vi "example.vi"() -> ()   [LabVIEW 2019]
panel:
  in  "Input Potentials":dbl[](array[numeric])
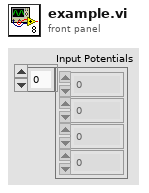
[diagram p1: front panel]
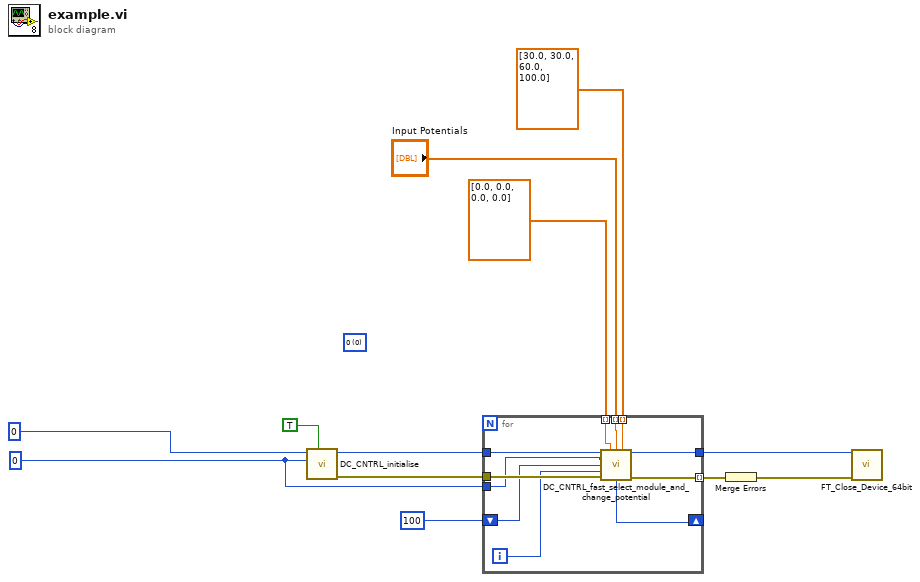
[diagram p0: block diagram]
diagram:
  (unwired) u16 0 items=["0", "1", "2", "3", "4", "5", "6", "7"] ("Current Module Number")
  w2 = 0 ("Box Number")
  n1 = call "DC_CNTRL_initialise.vi"("Check status?"=TRUE, "Box Number"=w2, "Device Index"=u32 0) -> ("error out"=w9:errorcluster, "Handle out"=w10:u64)  [unwired: 6 in, 1 out]
  n2 = for {
    tunnel: w10 -> [w23]
    tunnel: w9 -> [w22]
    tunnel: [w21] -> w8
    tunnel: [w20] -> w7 mode=indexing
    tunnel: "Input Potentials" -> [w18] mode=indexing
    tunnel: dbl[] [30.0, 30.0, 60.0, 100.0] ("Input Potentials") -> [w19] mode=indexing
    tunnel: dbl[] [0.0, 0.0, 0.0, 0.0] ("Input Potentials") -> [w17] mode=indexing
    tunnel: w2 -> [w16]
    shift-right: [w13] -> _
    shift-left: 100 -> [w15]
    i -> [w14]
    n3 = call "DC_CNTRL_fast_select_module_and_change_potential.vi"("Handle"=w23, "Current Potential (V)"=w17, "Target Potential (V)"=w18, "Max Potential (V)"=w19, "Box Number"=w16, "Current Module Number"=w15, "Desired Module Number"=w14, "error in (no error)"=w22) -> ("Handle out"=w21:u64, "Current Module Number Out"=w13:u16, "error out"=w20:errorcluster)  [unwired: 5 in]
  }
  n4 = Merge Errors(w7) -> (w6:errorcluster)
  n5 = call "FT_Close_Device_64bit.vi"("Handle"=w8, "error in (no error)"=w6) -> ()  [unwired: 12 in, 2 out]
